vi "CheckSettings.vi"(8 "error in (no error)":errorcluster, 11 "NHRDCPower in":refnum<class "NHRDCPower.lvclass">) -> (0 "error out":errorcluster, 3 "NHRDCPower out":refnum<class "NHRDCPower.lvclass">)   [LabVIEW 2018, in "AcPwrPlugins.lvlib" / "NHRDCPower.lvclass"]
doc: "This VI validates that all the configuration settings are accurate when the module is not updating on the fly."
uses:
  NHRDCPower.lvclass
  TypeDefs/CheckSettings.ctl
  <vilib>/Utility/error.llb/Error Cluster From Error Code.vi
  <vilib>/ErrorRing/Error Ring.xnode
  <instrlib>/NHRDCPowerModule/NHRDCPowerModule/NHRDCPowerModule.lvlib
panel:
  out "Check Settings Time":u32
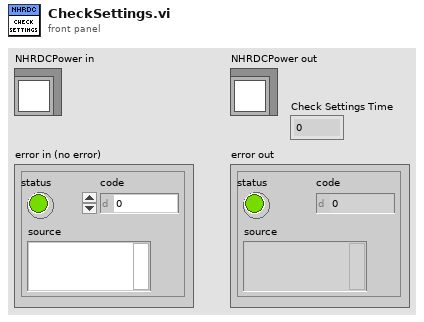
[diagram p1: front panel]
types:
  T1 = typedef "AcPwrPlugins.lvlib/NHRDCPower.lvclass/Modules.ctl" = cluster{"Handle":string, "Name":string, "id query (Yes)":bool, "reset device (Yes)":bool, "Connected":bool, "Initial Battery Detect Voltage (0)":dbl, "SafetySettings":cluster{"SetWatchDog?":bool, "Voltage (V)":dbl, "Current (A)":dbl, "Power (W)":dbl, "Voltage Delay (s)":dbl, "Current Delay (s)":dbl, "Power Delay (s)":dbl}, "Options String":string, "Aperture Time (s)":dbl, "operating state (Off)":i32, "OutputSettings":cluster{"Voltage (V)":dbl, "Current (A)":dbl, "Resistance (Ohms)":dbl, "Power (W)":dbl, "Enable Voltage":bool, "Enable Current":bool, "Enable Resistance":bool, "Enable Power":bool, "Macro After Step Delay  (s)":dbl, "Wait Value (V, A, W)":dbl, "Enable Wait":bool, "Wait on Value":i32}, "SlewRate":cluster{"Set Voltage Rate V/S":dbl, "Set Current Rate A/S":dbl, "Set Resistance Rate R/S":dbl, "Set Power Rate W/S":dbl}, "Macro":cluster{"Save Macro?":bool, "Load Macro From File?":bool, "Run Macro Continuously?":bool, "Use Macros?":bool, "Load Macro File Path":path, "Save Macro File Path":string}, "Regulation Gain (1=100%)":dbl, "UpdatingOntheFly":bool}[]
  T2 = typedef "AcPwrPlugins.lvlib/NHRDCPower.lvclass/CheckSettings.ctl" = enum16{"#ofOutputSettings", "RegulationGain", "Aperture", "Voltage", "Voltage Slew Rate", "Current", "Current Slew Rate", "Resistance", "Resistance Slew Rate", "Power", "Power Slew Rate", "RefreshTime"}
  T3 = cluster{"Set Voltage Rate V/S":dbl, "Set Current Rate A/S":dbl, "Set Resistance Rate R/S":dbl, "Set Power Rate W/S":dbl}
  T4 = cluster{"Voltage (V)":dbl, "Current (A)":dbl, "Resistance (Ohms)":dbl, "Power (W)":dbl, "Enable Voltage":bool, "Enable Current":bool, "Enable Resistance":bool, "Enable Power":bool, "Macro After Step Delay  (s)":dbl, "Wait Value (V, A, W)":dbl, "Enable Wait":bool, "Wait on Value":i32}
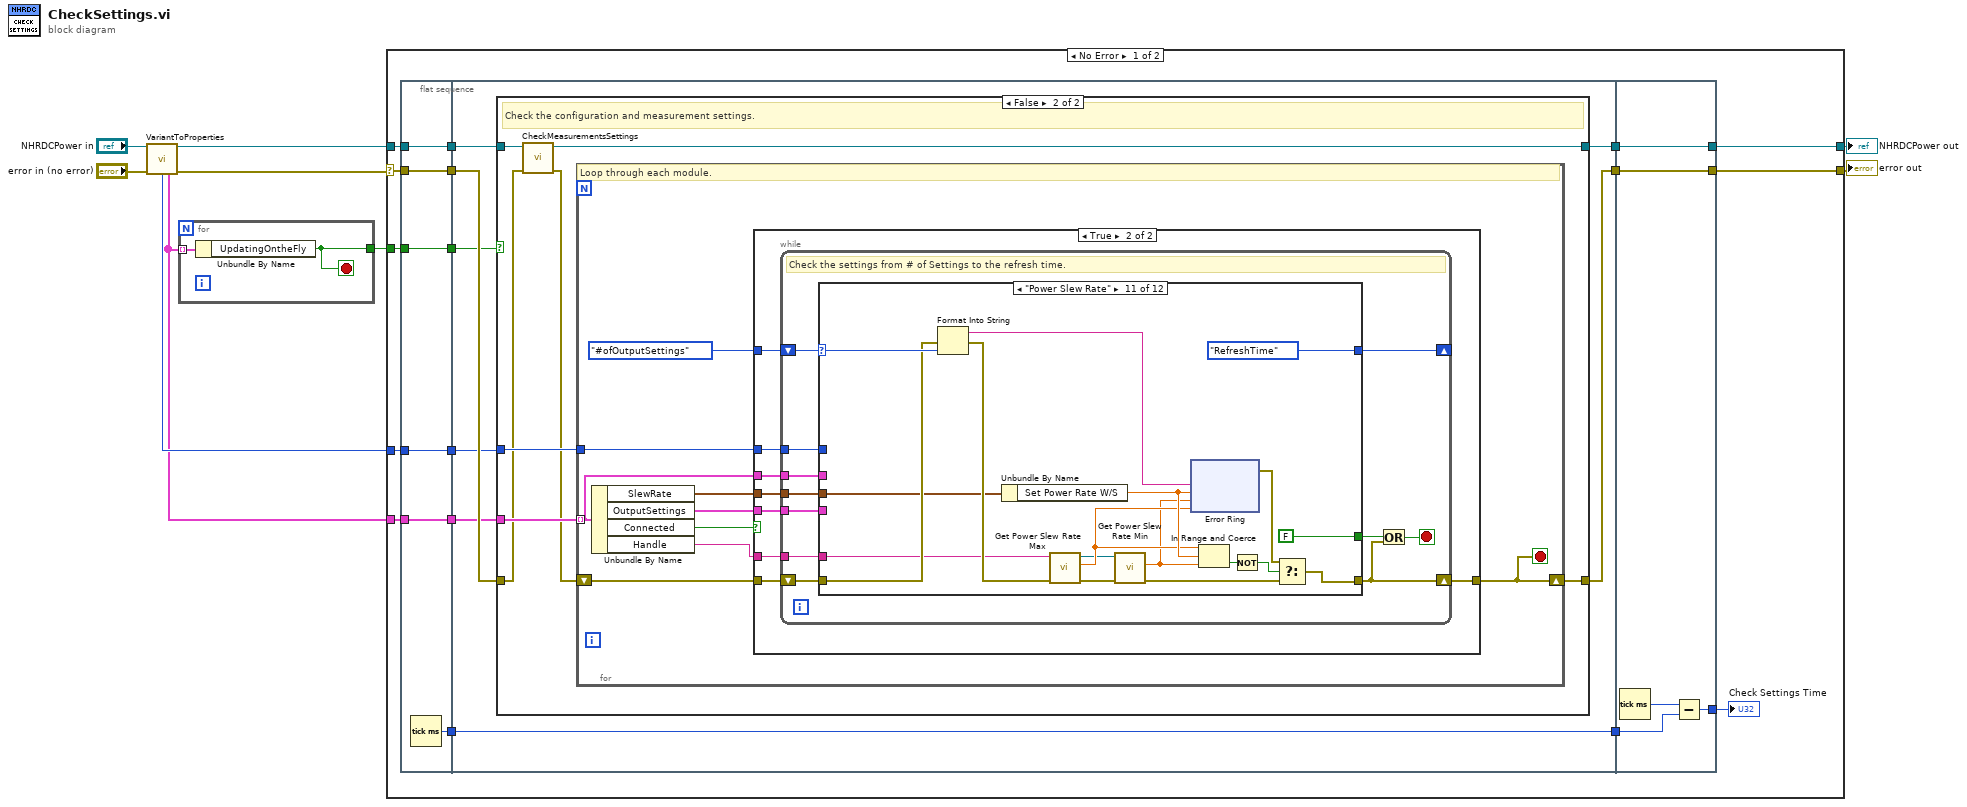
[diagram p0: block diagram]
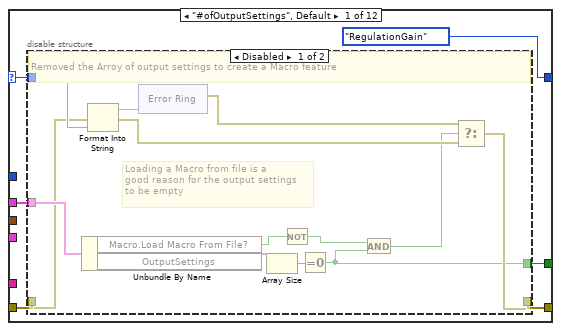
[diagram p4: hidden frame]
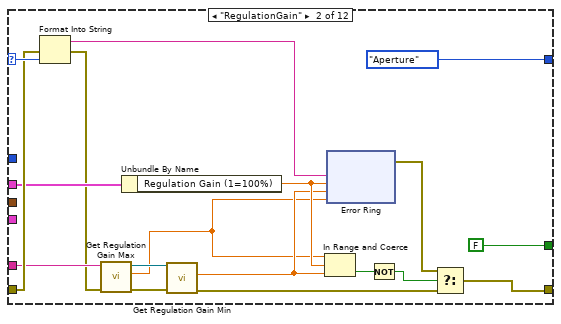
[diagram p6: hidden frame]
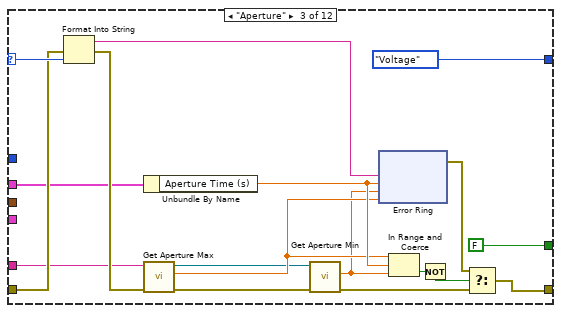
[diagram p7: hidden frame]
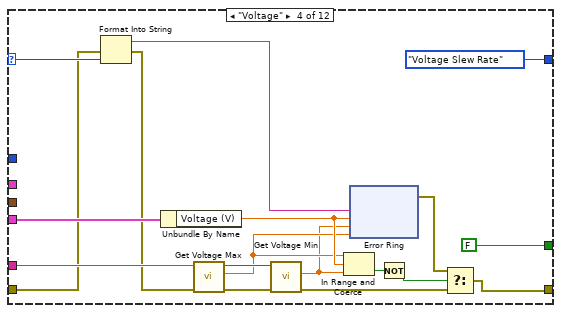
[diagram p8: hidden frame]
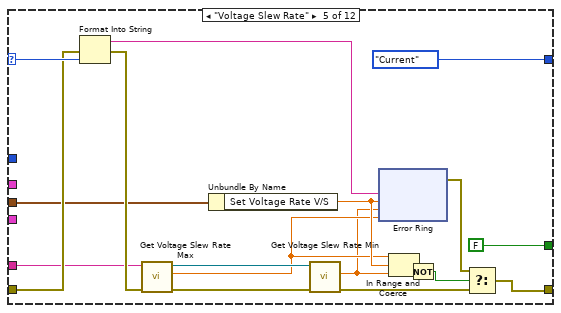
[diagram p9: hidden frame]
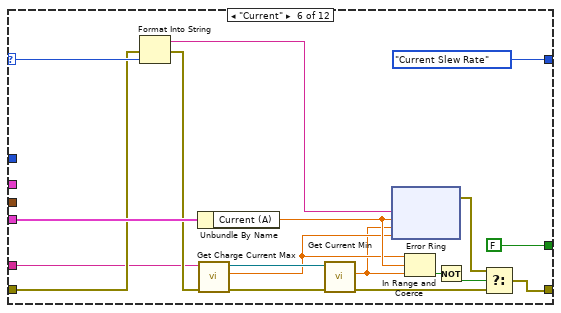
[diagram p10: hidden frame]
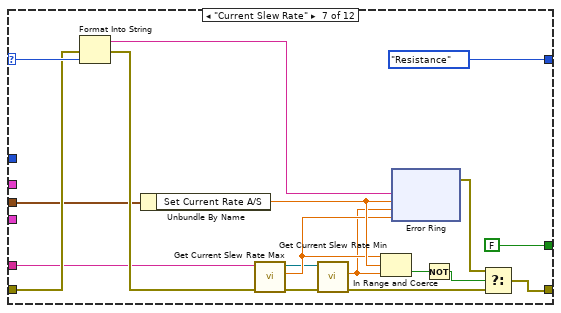
[diagram p11: hidden frame]
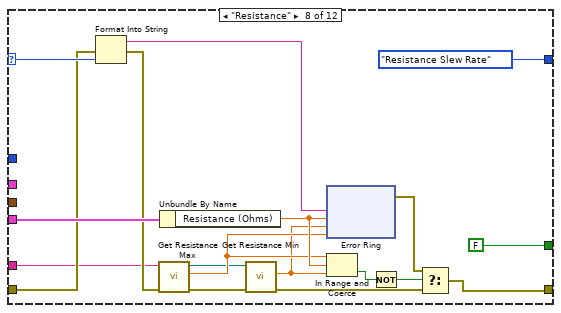
[diagram p12: hidden frame]
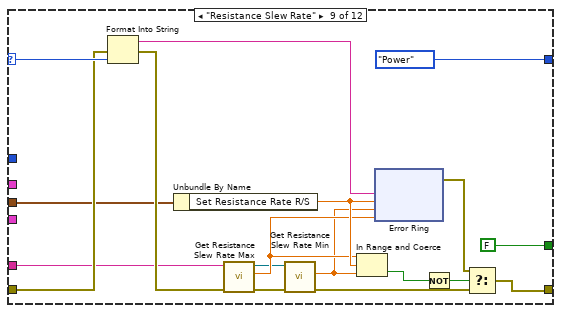
[diagram p13: hidden frame]
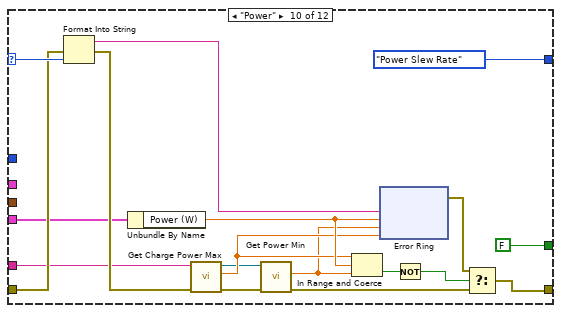
[diagram p14: hidden frame]
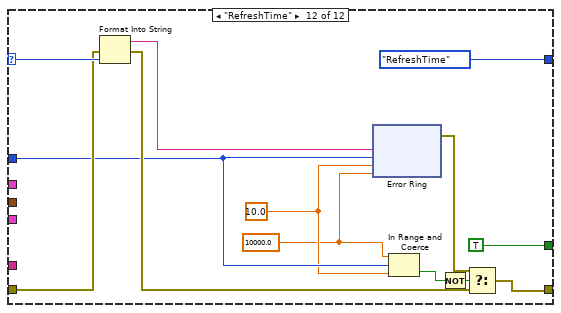
[diagram p15: hidden frame]
diagram:
  n1 = call "VariantToProperties.vi"("NHRDCPower in"="NHRDCPower in", "error in (no error)"="error in (no error)") -> ("NHRDCPower out"=w5:refnum<class "NHRDCPower.lvclass">, "Measurement Refresh Time (ms)"=w3:u32, "Modules"=w2:T1, "error out"=w6:errorcluster)  [unwired: 7 in, 3 out]
  n2 = for {
    tunnel: w2 -> [w11] mode=indexing
    tunnel: [w10] -> w1
    stop <- w10 stop-if-true
    n3 = Unbundle By Name(w11) -> ("UpdatingOntheFly"=w10:bool)
  }
  n4 = case shown="No Error" w6 {
    selector: w6 -> [w28 w417]
    tunnel: [w27 w417] -> w8
    tunnel: [w25 w416] -> w9
    tunnel: w5 -> [w26 w416]
    tunnel: w2 -> [w16 _]
    tunnel: w3 -> [w15 _]
    tunnel: w1 -> [w12 _]
    frame No Error {
      n5 = flat-sequence {
        tunnel: w26 -> [w33]
        tunnel: w28 -> [w34]
        tunnel: [w34] -> w24
        tunnel: [w33] -> w23
        tunnel: [w32] -> w20
        tunnel: [w31] -> w17
        tunnel: w16 -> [w31]
        tunnel: w15 -> [w30]
        tunnel: [w30] -> w14
        tunnel: [w29] -> w13
        tunnel: w12 -> [w29]
        tunnel: w24 -> [w41]
        tunnel: w23 -> [w36]
        tunnel: [w42] -> w22
        tunnel: [w35] -> w21
        tunnel: w20 -> [w40]
        tunnel: [w40] -> w19
        tunnel: w17 -> [w38]
        tunnel: w14 -> [w39]
        tunnel: w13 -> [w37]
        tunnel: [w414] -> w25
        tunnel: [w415] -> w27
        tunnel: w22 -> [w415]
        tunnel: w21 -> [w414]
        tunnel: w19 -> [w412]
        tunnel: [w411] -> w18
        frame #0 {
          n6 = Tick Count (ms)() -> (millisecond timer value=w32:u32)
        }
        frame #1 {
          n7 = case shown="False" w37 {
            tunnel: [w44 w51] -> w42
            tunnel: w41 -> [w44 w47]
            tunnel: w39 -> [_ w50]
            tunnel: w38 -> [_ w49]
            tunnel: w36 -> [w43 w48]
            tunnel: [w43 w46] -> w35
            frame True {
              # "If we are updating on the fly do not check any settings."
            }
            frame False {
              # "Check the configuration and measurement settings."
              n8 = call-dynamic "CheckMeasurementsSettings.vi"("error in (no error)"=w47, "NHRDCPower in"=w48) -> ("error out"=w45:errorcluster, "NHRDCPower out"=w46:refnum<class "NHRDCPower.lvclass">)  [unwired: 8 in]
              n9 = for {
                tunnel: w49 -> [w52] mode=indexing
                shift-right: [w60] -> w51
                shift-left: w45 -> [w55]
                tunnel: w50 -> [w53]
                stop <- w60 stop-if-true
                # "Loop through each module."
                n10 = Unbundle By Name(w52) -> ("SlewRate"=w56:T3, "OutputSettings"=w57:T4, "Connected"=w58:bool, "Handle"=w59:string)
                n11 = case shown="True" w58 {
                  tunnel: w55 -> [w61 w69]
                  tunnel: [w61 w66] -> w60
                  tunnel: w59 -> [_ w68]
                  tunnel: w57 -> [_ w67]
                  tunnel: w56 -> [_ w64]
                  tunnel: CheckSettings."#ofOutputSettings" ("CheckSettings Enum") -> [_ w65]
                  tunnel: w53 -> [_ w63]
                  tunnel: w52 -> [_ w62]
                  frame False {
                  }
                  frame True {
                    n12 = while {
                      tunnel: w68 -> [w79]
                      tunnel: w67 -> [w78]
                      shift-right: [w74] -> w66
                      shift-left: w69 -> [w80]
                      shift-right: [w73] -> _
                      shift-left: w65 -> [w77]
                      tunnel: w64 -> [w72]
                      tunnel: w63 -> [w71]
                      tunnel: w62 -> [w70]
                      stop <- w76 stop-if-true
                      # "Check the settings from # of Settings to the refresh time."
                      n13 = case shown="\"Power Slew Rate\"" w77 {
                        selector: w77 -> [w84 w120 w148 w169 w204 w231 w260 w287 w316 w344 w373 w396]
                        tunnel: w80 -> [w83 w119 w147 w168 w203 w230 w259 w286 w315 w343 w372 w395]
                        tunnel: w79 -> [_ w114 w143 w181 w200 w225 w256 w283 w312 w340 w369 _]
                        tunnel: w78 -> [_ _ _ w178 _ w237 _ w293 _ w338 _ _]
                        tunnel: [w82 w124 w152 w173 w208 w235 w264 w291 w320 w348 w377 w400] -> w74
                        tunnel: [w81 FALSE FALSE FALSE FALSE FALSE FALSE FALSE FALSE FALSE FALSE TRUE] -> w75
                        tunnel: [CheckSettings."RegulationGain" ("CheckSettings Enum") CheckSettings."Aperture" ("CheckSettings Enum") CheckSettings."Voltage" ("CheckSettings Enum") CheckSettings."Voltage Slew Rate" ("CheckSettings Enum") CheckSettings."Current" ("CheckSettings Enum") CheckSettings."Current Slew Rate" ("CheckSettings Enum") CheckSettings."Resistance" ("CheckSettings Enum") CheckSettings."Resistance Slew Rate" ("CheckSettings Enum") CheckSettings."Power" ("CheckSettings Enum") CheckSettings."Power Slew Rate" ("CheckSettings Enum") CheckSettings."RefreshTime" ("CheckSettings Enum") CheckSettings."RefreshTime" ("CheckSettings Enum")] -> w73
                        tunnel: w72 -> [_ _ _ _ w193 _ w254 _ w310 _ w367 _]
                        tunnel: w71 -> [_ _ _ _ _ _ _ _ _ _ _ w390]
                        tunnel: w70 -> [w85 w115 w136 _ _ _ _ _ _ _ _ _]
                        frame "#ofOutputSettings", Default {
                          n14 = disable-structure shown="Disabled" {
                            disable-tunnel: w85 -> [w99 _]
                            disable-tunnel: w84 -> [w96 _]
                            disable-tunnel: w83 -> [w95 w107]
                            disable-tunnel: [w91 w107] -> w82
                            disable-tunnel: [w90 _] -> w81
                            frame Disabled {
                              # "Loading a Macro from file is a \ngood reason for the output settings\nto be empty"
                              # "Removed the Arroy of output settings to create a Macro feature"
                              n15 = Unbundle By Name(w99) -> ("Macro.Load Macro From File?"=w87:bool, "OutputSettings"=w98:T4)
                              n16 = Format Into String(error in=w95, w96) -> (resulting string=w93:string, error out=w94:errorcluster)  [unwired: 2 in]
                              n17 = xnode "Error Ring"("parameter 0"=w93) -> ("error out"=w92:errorcluster)
                              n18 = Array Size(array=w98) -> (size(s)=w97:i32)
                              n19 = Not(x=w87) -> (.not. x?=w88:bool)
                              n20 = Equal To 0?(x=w97) -> (x = 0?=w90:bool)
                              n21 = And(x=w88, y=w90) -> (x .and. y?=w89:bool)
                              n22 = Select(t=w92, s=w89, f=w94) -> (s? t:f=w91:errorcluster)
                            }
                            frame Enabled {
                            }
                          }
                        }
                        frame "RegulationGain" {
                          n23 = Format Into String(error in=w119, w120) -> (resulting string=w118:string, error out=w109:errorcluster)  [unwired: 2 in]
                          n24 = call <instrlib>:"Get Regulation Gain Max.vi"("error in (no error)"=w109, "instrument handle"=w114) -> ("error out"=w112:errorcluster, "maximum gain"=w108:sgl, "instrument handle out"=w113:refnum<visa-resource-name>)  [unwired: 7 in]
                          n25 = Unbundle By Name(w115) -> ("Regulation Gain (1=100%)"=w125:dbl)
                          n26 = call <instrlib>:"Get Regulation Gain Min.vi"("error in (no error)"=w112, "instrument handle"=w113) -> ("error out"=w111:errorcluster, "minimum gain"=w110:sgl)  [unwired: 7 in, 1 out]
                          n27 = In Range and Coerce(upper limit=w108, x=w125, lower limit=w110) -> (In Range?=w122:bool)  [unwired: 1 out]
                          n28 = xnode "Error Ring"("parameter 0"=w118, "parameter 1"=w125, "parameter 2"=w110, "parameter 3"=w108) -> ("error out"=w123:errorcluster)
                          n29 = Not(x=w122) -> (.not. x?=w116:bool)
                          n30 = Select(t=w123, s=w116, f=w111) -> (s? t:f=w124:errorcluster)
                        }
                        frame "Aperture" {
                          n31 = Format Into String(error in=w147, w148) -> (resulting string=w145:string, error out=w146:errorcluster)  [unwired: 2 in]
                          n32 = Unbundle By Name(w136) -> ("Aperture Time (s)"=w153:dbl)
                          n33 = call <instrlib>:"Get Aperture Max.vi"("error in (no error)"=w146, "instrument handle"=w143) -> ("error out"=w144:errorcluster, "maximum aperture"=w142:sgl, "instrument handle out"=w141:refnum<visa-resource-name>)  [unwired: 7 in]
                          n34 = call <instrlib>:"Get Aperture Min.vi"("error in (no error)"=w144, "instrument handle"=w141) -> ("error out"=w139:errorcluster, "minimum aperture"=w140:sgl)  [unwired: 7 in, 1 out]
                          n35 = xnode "Error Ring"("parameter 0"=w145, "parameter 1"=w153, "parameter 2"=w140, "parameter 3"=w142) -> ("error out"=w151:errorcluster)
                          n36 = In Range and Coerce(upper limit=w142, x=w153, lower limit=w140) -> (In Range?=w150:bool)  [unwired: 1 out]
                          n37 = Not(x=w150) -> (.not. x?=w137:bool)
                          n38 = Select(t=w151, s=w137, f=w139) -> (s? t:f=w152:errorcluster)
                        }
                        frame "Voltage" {
                          n39 = Format Into String(error in=w168, w169) -> (resulting string=w166:string, error out=w167:errorcluster)  [unwired: 2 in]
                          n40 = Unbundle By Name(w178) -> ("Voltage (V)"=w177:dbl)
                          n41 = call <instrlib>:"Get Voltage Max.vi"("error in (no error)"=w167, "instrument handle"=w181) -> ("error out"=w179:errorcluster, "maximum voltage"=w176:sgl, "instrument handle out"=w180:refnum<visa-resource-name>)  [unwired: 7 in]
                          n42 = call <instrlib>:"Get Voltage Min.vi"("error in (no error)"=w179, "instrument handle"=w180) -> ("error out"=w174:errorcluster, "minimum voltage"=w175:sgl)  [unwired: 7 in, 1 out]
                          n43 = In Range and Coerce(upper limit=w176, x=w177, lower limit=w175) -> (In Range?=w171:bool)  [unwired: 1 out]
                          n44 = xnode "Error Ring"("parameter 0"=w166, "parameter 1"=w177, "parameter 2"=w175, "parameter 3"=w176) -> ("error out"=w172:errorcluster)
                          n45 = Not(x=w171) -> (.not. x?=w164:bool)
                          n46 = Select(t=w172, s=w164, f=w174) -> (s? t:f=w173:errorcluster)
                        }
                        frame "Voltage Slew Rate" {
                          n47 = Format Into String(error in=w203, w204) -> (resulting string=w201:string, error out=w202:errorcluster)  [unwired: 2 in]
                          n48 = call <instrlib>:"Get Voltage Slew Rate Max.vi"("error in (no error)"=w202, "instrument handle"=w200) -> ("error out"=w198:errorcluster, "maximum voltage slew rate"=w195:sgl, "instrument handle out"=w196:refnum<visa-resource-name>)  [unwired: 7 in]
                          n49 = Unbundle By Name(w193) -> ("Set Voltage Rate V/S"=w209:dbl)
                          n50 = call <instrlib>:"Get Voltage Slew Rate Min.vi"("error in (no error)"=w198, "instrument handle"=w196) -> ("error out"=w197:errorcluster, "minimum voltage slew rate"=w194:sgl)  [unwired: 7 in, 1 out]
                          n51 = xnode "Error Ring"("parameter 0"=w201, "parameter 1"=w209, "parameter 2"=w194, "parameter 3"=w195) -> ("error out"=w207:errorcluster)
                          n52 = In Range and Coerce(upper limit=w195, x=w209, lower limit=w194) -> (In Range?=w206:bool)  [unwired: 1 out]
                          n53 = Not(x=w206) -> (.not. x?=w192:bool)
                          n54 = Select(t=w207, s=w192, f=w197) -> (s? t:f=w208:errorcluster)
                        }
                        frame "Current" {
                          n55 = Format Into String(error in=w230, w231) -> (resulting string=w228:string, error out=w229:errorcluster)  [unwired: 2 in]
                          n56 = Unbundle By Name(w237) -> ("Current (A)"=w236:dbl)
                          n57 = call <instrlib>:"Get Charge Current Max.vi"("error in (no error)"=w229, "instrument handle"=w225) -> ("error out"=w226:errorcluster, "charge current max"=w223:sgl, "instrument handle out"=w224:refnum<visa-resource-name>)  [unwired: 7 in]
                          n58 = call <instrlib>:"Get Current Min.vi"("error in (no error)"=w226, "instrument handle"=w224) -> ("error out"=w227:errorcluster, "minimum current"=w222:sgl)  [unwired: 7 in, 1 out]
                          n59 = xnode "Error Ring"("parameter 0"=w228, "parameter 1"=w236, "parameter 2"=w222, "parameter 3"=w223) -> ("error out"=w234:errorcluster)
                          n60 = In Range and Coerce(upper limit=w223, x=w236, lower limit=w222) -> (In Range?=w233:bool)  [unwired: 1 out]
                          n61 = Not(x=w233) -> (.not. x?=w220:bool)
                          n62 = Select(t=w234, s=w220, f=w227) -> (s? t:f=w235:errorcluster)
                        }
                        frame "Current Slew Rate" {
                          n63 = Format Into String(error in=w259, w260) -> (resulting string=w257:string, error out=w258:errorcluster)  [unwired: 2 in]
                          n64 = Unbundle By Name(w254) -> ("Set Current Rate A/S"=w265:dbl)
                          n65 = call <instrlib>:"Get Current Slew Rate Max.vi"("error in (no error)"=w258, "instrument handle"=w256) -> ("error out"=w253:errorcluster, "maximum current slew rate"=w252:sgl, "instrument handle out"=w250:refnum<visa-resource-name>)  [unwired: 7 in]
                          n66 = call <instrlib>:"Get Current Slew Rate Min.vi"("error in (no error)"=w253, "instrument handle"=w250) -> ("error out"=w251:errorcluster, "minimum current slew rate"=w249:sgl)  [unwired: 7 in, 1 out]
                          n67 = In Range and Coerce(upper limit=w252, x=w265, lower limit=w249) -> (In Range?=w262:bool)  [unwired: 1 out]
                          n68 = xnode "Error Ring"("parameter 0"=w257, "parameter 1"=w265, "parameter 2"=w249, "parameter 3"=w252) -> ("error out"=w263:errorcluster)
                          n69 = Not(x=w262) -> (.not. x?=w248:bool)
                          n70 = Select(t=w263, s=w248, f=w251) -> (s? t:f=w264:errorcluster)
                        }
                        frame "Resistance" {
                          n71 = Format Into String(error in=w286, w287) -> (resulting string=w284:string, error out=w285:errorcluster)  [unwired: 2 in]
                          n72 = call <instrlib>:"Get Resistance Max.vi"("error in (no error)"=w285, "instrument handle"=w283) -> ("error out"=w282:errorcluster, "maximum resistance"=w281:sgl, "instrument handle out"=w279:refnum<visa-resource-name>)  [unwired: 7 in]
                          n73 = Unbundle By Name(w293) -> ("Resistance (Ohms)"=w292:dbl)
                          n74 = call <instrlib>:"Get Resistance Min.vi"("error in (no error)"=w282, "instrument handle"=w279) -> ("error out"=w280:errorcluster, "minimum resistance"=w278:sgl)  [unwired: 7 in, 1 out]
                          n75 = xnode "Error Ring"("parameter 0"=w284, "parameter 1"=w292, "parameter 2"=w278, "parameter 3"=w281) -> ("error out"=w290:errorcluster)
                          n76 = In Range and Coerce(upper limit=w281, x=w292, lower limit=w278) -> (In Range?=w289:bool)  [unwired: 1 out]
                          n77 = Not(x=w289) -> (.not. x?=w276:bool)
                          n78 = Select(t=w290, s=w276, f=w280) -> (s? t:f=w291:errorcluster)
                        }
                        frame "Resistance Slew Rate" {
                          n79 = Format Into String(error in=w315, w316) -> (resulting string=w313:string, error out=w314:errorcluster)  [unwired: 2 in]
                          n80 = Unbundle By Name(w310) -> ("Set Resistance Rate R/S"=w321:dbl)
                          n81 = call <instrlib>:"Get Resistance Slew Rate Max.vi"("error in (no error)"=w314, "instrument handle"=w312) -> ("error out"=w309:errorcluster, "maximum resistance slew rate"=w308:sgl, "instrument handle out"=w305:refnum<visa-resource-name>)  [unwired: 7 in]
                          n82 = call <instrlib>:"Get Resistance Slew Rate Min.vi"("error in (no error)"=w309, "instrument handle"=w305) -> ("error out"=w307:errorcluster, "minimum resistance slew rate"=w306:sgl)  [unwired: 7 in, 1 out]
                          n83 = In Range and Coerce(upper limit=w308, x=w321, lower limit=w306) -> (In Range?=w318:bool)  [unwired: 1 out]
                          n84 = xnode "Error Ring"("parameter 0"=w313, "parameter 1"=w321, "parameter 2"=w306, "parameter 3"=w308) -> ("error out"=w319:errorcluster)
                          n85 = Not(x=w318) -> (.not. x?=w304:bool)
                          n86 = Select(t=w319, s=w304, f=w307) -> (s? t:f=w320:errorcluster)
                        }
                        frame "Power" {
                          n87 = Format Into String(error in=w343, w344) -> (resulting string=w341:string, error out=w342:errorcluster)  [unwired: 2 in]
                          n88 = Unbundle By Name(w338) -> ("Power (W)"=w349:dbl)
                          n89 = call <instrlib>:"Get Charge Power Max.vi"("error in (no error)"=w342, "instrument handle"=w340) -> ("error out"=w337:errorcluster, "charge power max"=w336:sgl, "instrument handle out"=w333:refnum<visa-resource-name>)  [unwired: 7 in]
                          n90 = call <instrlib>:"Get Power Min.vi"("error in (no error)"=w337, "instrument handle"=w333) -> ("error out"=w335:errorcluster, "minimum power"=w334:sgl)  [unwired: 7 in, 1 out]
                          n91 = In Range and Coerce(upper limit=w336, x=w349, lower limit=w334) -> (In Range?=w346:bool)  [unwired: 1 out]
                          n92 = xnode "Error Ring"("parameter 0"=w341, "parameter 1"=w349, "parameter 2"=w334, "parameter 3"=w336) -> ("error out"=w347:errorcluster)
                          n93 = Not(x=w346) -> (.not. x?=w332:bool)
                          n94 = Select(t=w347, s=w332, f=w335) -> (s? t:f=w348:errorcluster)
                        }
                        frame "Power Slew Rate" {
                          n95 = Format Into String(error in=w372, w373) -> (resulting string=w370:string, error out=w371:errorcluster)  [unwired: 2 in]
                          n96 = Unbundle By Name(w367) -> ("Set Power Rate W/S"=w366:dbl)
                          n97 = call <instrlib>:"Get Power Slew Rate Max.vi"("error in (no error)"=w371, "instrument handle"=w369) -> ("error out"=w365:errorcluster, "maximum power slew rate"=w364:sgl, "instrument handle out"=w362:refnum<visa-resource-name>)  [unwired: 7 in]
                          n98 = call <instrlib>:"Get Power Slew Rate Min.vi"("error in (no error)"=w365, "instrument handle"=w362) -> ("error out"=w363:errorcluster, "minimum power slew rate"=w361:sgl)  [unwired: 7 in, 1 out]
                          n99 = xnode "Error Ring"("parameter 0"=w370, "parameter 1"=w366, "parameter 2"=w361, "parameter 3"=w364) -> ("error out"=w376:errorcluster)
                          n100 = In Range and Coerce(upper limit=w364, x=w366, lower limit=w361) -> (In Range?=w375:bool)  [unwired: 1 out]
                          n101 = Not(x=w375) -> (.not. x?=w360:bool)
                          n102 = Select(t=w376, s=w360, f=w363) -> (s? t:f=w377:errorcluster)
                        }
                        frame "RefreshTime" {
                          w388 = 10000.0 ("parameter 2")
                          w389 = 10.0 ("parameter 2")
                          n103 = Format Into String(error in=w395, w396) -> (resulting string=w393:string, error out=w394:errorcluster)  [unwired: 2 in]
                          n104 = xnode "Error Ring"("parameter 0"=w393, "parameter 1"=w390, "parameter 2"=w389, "parameter 3"=w388) -> ("error out"=w399:errorcluster)
                          n105 = In Range and Coerce(upper limit=w388, x=w390, lower limit=w389) -> (In Range?=w398:bool)  [unwired: 1 out]
                          n106 = Not(x=w398) -> (.not. x?=w391:bool)
                          n107 = Select(t=w399, s=w391, f=w394) -> (s? t:f=w400:errorcluster)
                        }
                      }
                      n108 = Or(x=w75, y=w74) -> (x .or. y?=w76:bool)
                    }
                  }
                }
              }
            }
          }
        }
        frame #2 {
          n109 = Tick Count (ms)() -> (millisecond timer value=w413:u32)
          n110 = Subtract(x=w413, y=w412) -> (x-y=w411:u32)
        }
      }
      "Check Settings Time" <- w18
    }
    frame Error {
    }
  }
  "error out" <- w8
  "NHRDCPower out" <- w9
